vi "Read Measurement Memory 1.vi"(8 "error in (no error)":errorcluster, 9 "Enable Wait (F: Disable)":bool, 10 "Reading Count (1)":dbl=1.0, 11 "VISA resource name":refnum<visa-resource-name>) -> (0 "error out":errorcluster, 2 "Read Result":dbl[](array[numeric]), 3 "VISA resource name out":refnum<visa-resource-name>)   [LabVIEW 2015, in "Agilent 3446X Series1.lvlib"]
doc: "Reads the measurement memory."
uses:
  Agilent 3446X Series1.lvlib
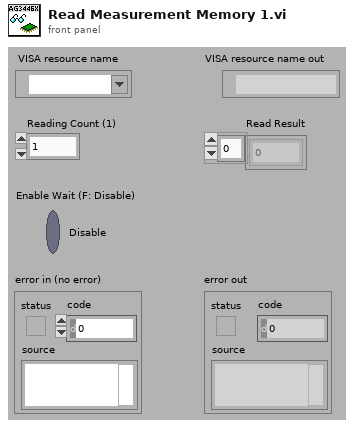
[diagram p1: front panel]
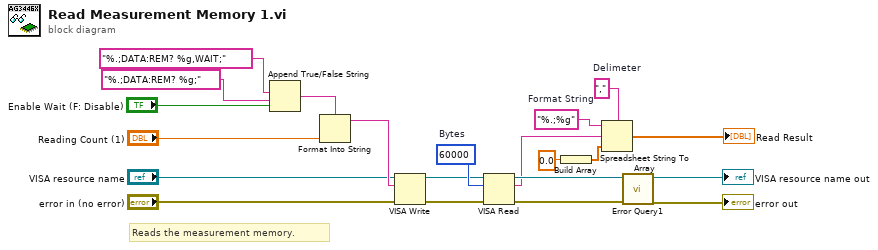
[diagram p0: block diagram]
diagram:
  w9 = ","  # Delimeter
  w10 = "%.;%g"  # Format String
  w15 = u32 60000  # Bytes
  # "Reads the measurement memory."
  n1 = Append True/False String(1:"Enable Wait (F: Disable)", 2:"%.;DATA:REM? %g;", 3:"%.;DATA:REM? %g,WAIT;") -> (0:w4:string)  [unwired: 1 in]
  n2 = Format Into String(format string=w4, "Reading Count (1)") -> (resulting string=w20:string)  [unwired: 2 in, 1 out]
  n3 = VISA Write(VISA resource name="VISA resource name", write buffer=w20, error in (no error)="error in (no error)") -> (VISA resource name out=w14:refnum<visa-resource-name>, error out=w13:errorcluster)  [unwired: 1 out]
  n4 = VISA Read(VISA resource name=w14, byte count=w15, error in (no error)=w13) -> (VISA resource name out=w12:refnum<visa-resource-name>, read buffer=w6:string, error out=w11:errorcluster)  [unwired: 1 out]
  n5 = Build Array(0.0) -> (w7:dbl[])
  n6 = Spreadsheet String To Array(delimiter (Tab)=w9, format string=w10, spreadsheet string=w6, array type (2D Dbl)=w7) -> (array=→"Read Result":dbl[])
  n7 = call "Error Query1.vi"("error in (no error)"=w11, "VISA resource name"=w12) -> ("error out"=→"error out":errorcluster, "VISA resource name out"=→"VISA resource name out":refnum<visa-resource-name>)  [unwired: 8 out]
